vi "On Compile Action VI Name.vi"(11 "CD Template in":refnum<class "NIVS_PPL_Inline HW Interface (Inline-Async).lvclass">) -> (2 "On Compile Action VI Name":string)   [LabVIEW 2020, in "NIVS_PPL_Inline HW Interface (Inline-Async).lvclass"]
uses:
  NIVS_PPL_Inline HW Interface (Inline-Async).lvclass
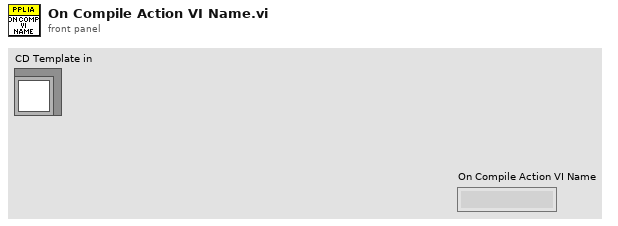
[diagram p1: front panel]
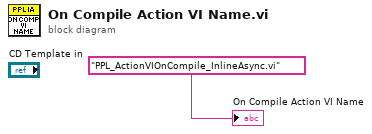
[diagram p0: block diagram]
diagram:
  "On Compile Action VI Name" <- "PPL_ActionVIOnCompile_InlineAsync.vi" ("On Compile Action VI Name")
